vi "oax_Check Tacho Channel Selection (DSA).vi"(8 "error in (no error)":errorcluster, 9 "tachometer channel":tag, 10 "tacho type":enum16{"Analog Tacho", "Digital Tacho"}(ring), 11 "DAQ Config":T1 {"pregain" format="%.2f"; "IEPE" items=["On", "Off", "None"]; "coupling" items=["DC", "AC"]; "engineering units" items=["custom..."=0, "V"=1, "A"=21, "C"=30, "pC"=31, "s"=32, "-"=29, "Pa"=2, "N"=20, "g"=3, "m/s^2"=4, "m/s"=5, "m"=6, "mm/s"=12, "mm"=13, "micron/s"=14, "micron"=15, "in/s^2"=7, "in/s"=8, "in"=9, "mil/s"=10, "mil"=11, "rad/s^2"=16, "rad/s"=17, "rad"=18, "deg/s^2"=26, "deg/s"=27, "deg"=28, "RPM"=22, "cycle/s^2"=23, "Hz"=24, "cycle"=25, "strain"=19]; "sensor sensitivity (mV/EU)" format="%.2f"; "dB reference" format="%.1e"}) -> (0 "error out":errorcluster, 1 "tachometer channel selected":tag, 2 "dul tacho type":enum16{"Analog Tacho", "Digital Tacho"}(ring), 3 "tacho channel index":i32)   [LabVIEW 2017]
uses:
  <vilib>/addons/Sound and Vibration/Order Analysis/Example Support/sub VIs/OAXML_DSA DAQ Config.ctl
  <vilib>/addons/_NISVFA/_Shared subVIs/Controls/svc_Engineering Units Text Ring.ctl
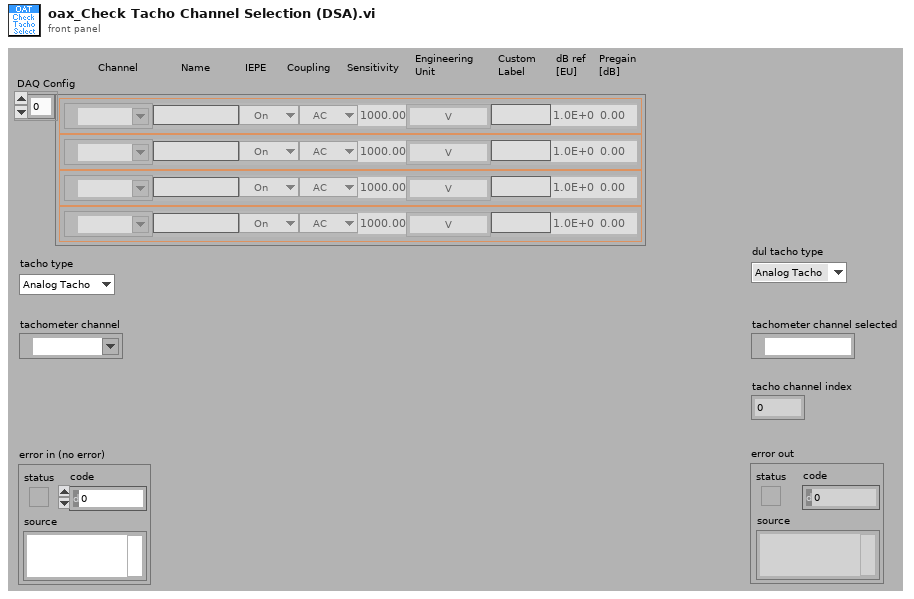
[diagram p1: front panel]
types:
  T1 = typedef "OAXML_DSA DAQ Config.ctl" = cluster{"name":string, "channel":tag, "coupling":u16, "dB reference":sgl, "sensor sensitivity (mV/EU)":dbl, "engineering units":T2, "IEPE":u16, "custom label":string, "pregain":sgl}[]
  T2 = typedef "svc_Engineering Units Text Ring.ctl" = u16
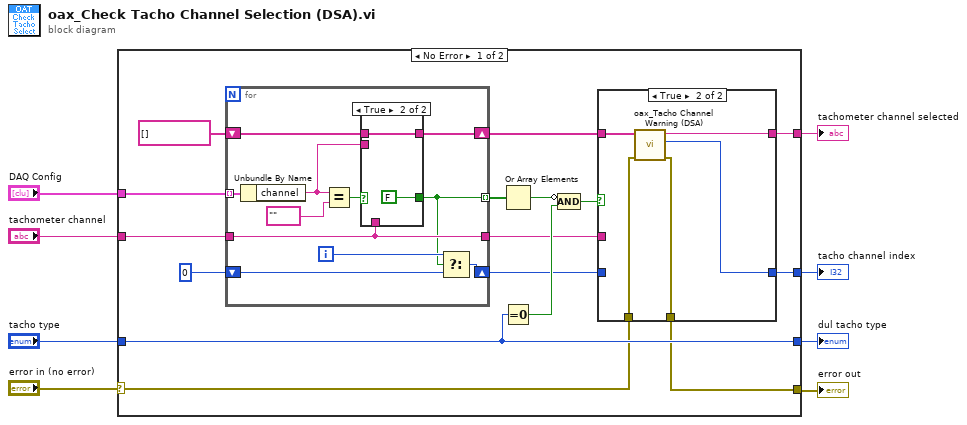
[diagram p0: block diagram]
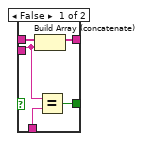
[diagram p3: hidden frame]
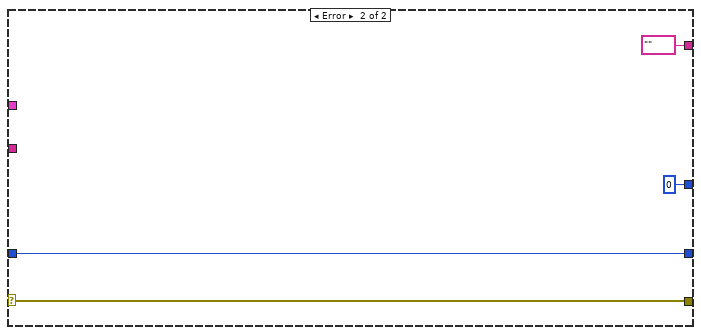
[diagram p4: hidden frame]
diagram:
  n1 = case shown="No Error" "error in (no error)" {
    selector: "error in (no error)" -> [w12 w52]
    tunnel: "DAQ Config" -> [w24 _]
    tunnel: "tachometer channel" -> [w23 _]
    tunnel: "tacho type" -> [w13 w54]
    tunnel: [w16 0] -> w5
    tunnel: [w13 w54] -> w4
    tunnel: [w11 w52] -> w2
    tunnel: [w10 tag "" ("tachometer channel")] -> w1
    frame No Error {
      n2 = for {
        tunnel: w24 -> [w43] mode=indexing
        tunnel: w23 -> [w36]
        tunnel: [w35] -> w22 mode=indexing
        shift-right: [w40] -> w17
        shift-left: 0 -> [w41]
        shift-right: [w37] -> w14
        shift-left: tag[] [] -> [w38]
        tunnel: [w36] -> w9
        i -> [w42]
        n3 = Unbundle By Name(w43) -> ("channel"=w34:tag)
        n4 = Equal?(x=w34, y=tag "" ("channel")) -> (x = y?=w39:bool)
        n5 = case shown="True" w39 {
          tunnel: w38 -> [w48 w50]
          tunnel: [w47 w50] -> w37
          tunnel: w34 -> [w46 _]
          tunnel: w36 -> [w45 _]
          tunnel: [w44 FALSE] -> w35
          frame False {
            n6 = Build Array (concatenate)(w48, w46) -> (w47:tag[])
            n7 = Equal?(x=w46, y=w45) -> (x = y?=w44:bool)
          }
          frame True {
          }
        }
        n8 = Select(t=w42, s=w35, f=w41) -> (s? t:f=w40:i32)
      }
      n9 = Or Array Elements(Boolean array=w22) -> (logical OR=w21:bool)
      n10 = Equal To 0?(x=w13) -> (x = 0?=w20:bool)
      n11 = Compound Arithmetic op=AND(invert w21, w20) -> (w18:bool)
      n12 = case shown="True" w18 {
        tunnel: w17 -> [w27 _]
        tunnel: [w27 w29] -> w16
        tunnel: w14 -> [_ w32]
        tunnel: w12 -> [w26 w31]
        tunnel: [w26 w30] -> w11
        tunnel: [w25 w28] -> w10
        tunnel: w9 -> [w25 _]
        frame False {
        }
        frame True {
          n13 = call <vilib>:"oax_Tacho Channel Warning (DSA).vi"("error in (no error)"=w31, "legal channels"=w32) -> ("error out"=w30:errorcluster, "tacho channel index"=w29:i32, "tachometer channel"=w28:tag)  [unwired: 7 in]
        }
      }
    }
    frame Error {
    }
  }
  "dul tacho type" <- w4
  "tacho channel index" <- w5
  "error out" <- w2
  "tachometer channel selected" <- w1
